vi "CalculateSpeed.vi"(8 "error in (no error)":errorcluster, 11 "Pulse Positions":dbl[](array[numeric])) -> (0 "error out":errorcluster, 2 "Speed (RPM)":dbl)   [LabVIEW 2017, in "AnalysisHelper.lvlib"]
uses:
  <vilib>/addons/InsightCM/Utilities/Analysis/Shared/AnalysisHelper.lvlib
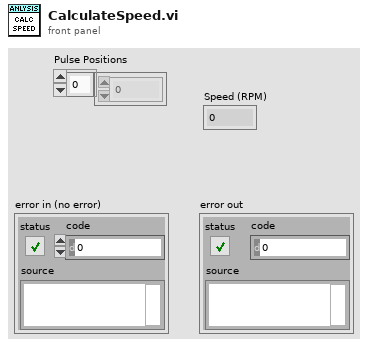
[diagram p1: front panel]
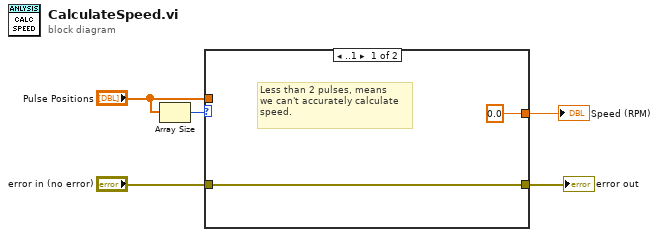
[diagram p0: block diagram]
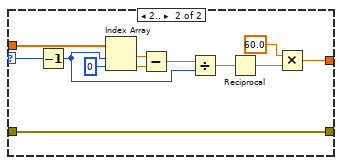
[diagram p2: hidden frame]
diagram:
  n1 = Array Size(array="Pulse Positions") -> (size(s)=w5:i32)
  n2 = case shown="..1" w5 {
    selector: w5 -> [_ w9]
    tunnel: [sgl 0.0 w19] -> w1
    tunnel: "Pulse Positions" -> [_ w14]
    tunnel: [w6 w8] -> w3
    tunnel: "error in (no error)" -> [w6 w8]
    frame ..1 {
      # "Less than 2 pulses, means\nwe can't accurately calculate\nspeed."
    }
    frame 2.. {
      n3 = Decrement(x=w9) -> (x-1=w17:i32)
      n4 = Index Array(array=w14, index #1=w17, index #2=0 ("index")) -> (element #1=w15:dbl, element #2=w12:dbl)
      n5 = Subtract(x=w15, y=w12) -> (x-y=w16:dbl)
      n6 = Divide(x=w16, y=w17) -> (x/y=w11:dbl)
      n7 = Reciprocal(x=w11) -> (1/x=w10:dbl)
      n8 = Multiply(x=sgl 60.0, y=w10) -> (x*y=w19:dbl)
    }
  }
  "Speed (RPM)" <- w1
  "error out" <- w3
